vi "Configure controller.vi"(2 "Ti (s)":sgl=0.1, 3 "Kp":sgl=0.035, 4 "RPM":sgl(knob) min=-1000 max=1000 scale=-1000.0..1000.0, 5 "Set RPM only (else full config.)":bool) -> (0 "error out":errorcluster)   [LabVIEW 2015]
uses:
  Arduino_common/Arduino_comms_Global.vi
panel:
  in  "Device index":i32=1
  in  "Reset":bool
  in  "Control system configuration":enum32{"Encoder", "Motor", "RPM", "PID"}(tab)=enum."PID"
  in  "Encoder PPR":u16=256
  in  "Encoder x1/x2/x4":u8(ring)=1 items=["1"=1, "2"=2, "4"=4]
  in  "Vmotor_max":sgl=6.0
  in  "Vmotor_min":sgl=-6.0
  in  "Gearbox ratio (shaft : motor)":sgl=0.24561404
  in  "RPM_max":sgl=1000.0
  in  "RPM_min":sgl=-1000.0
  in  "RPM_tol":sgl
  in  "Td (s)":sgl
  out "Bytes sent":u32
  out "Write buffer":string
  # "Paul Nathan, 03/08/2013"
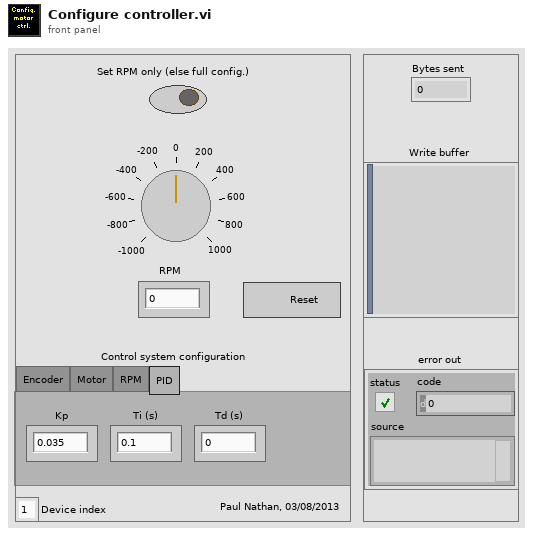
[diagram p1: front panel]
types:
  T1 = typedef "Arduino Config & resource typedef.ctl" = cluster{"VISA resource name":refnum<visa-resource-name>, "baud rate (bps)":u32, "timeout (ms)":u32, "data bits":u16, "parity":enum16{"None", "Odd", "Even", "Mark", "Space"}, "stop bits (10: 1 bit)":u16, "flow control":u16, "termination char (hex)":u8, "Enable Termination Char":bool, "byte count":u32, "Resource locked?":bool}
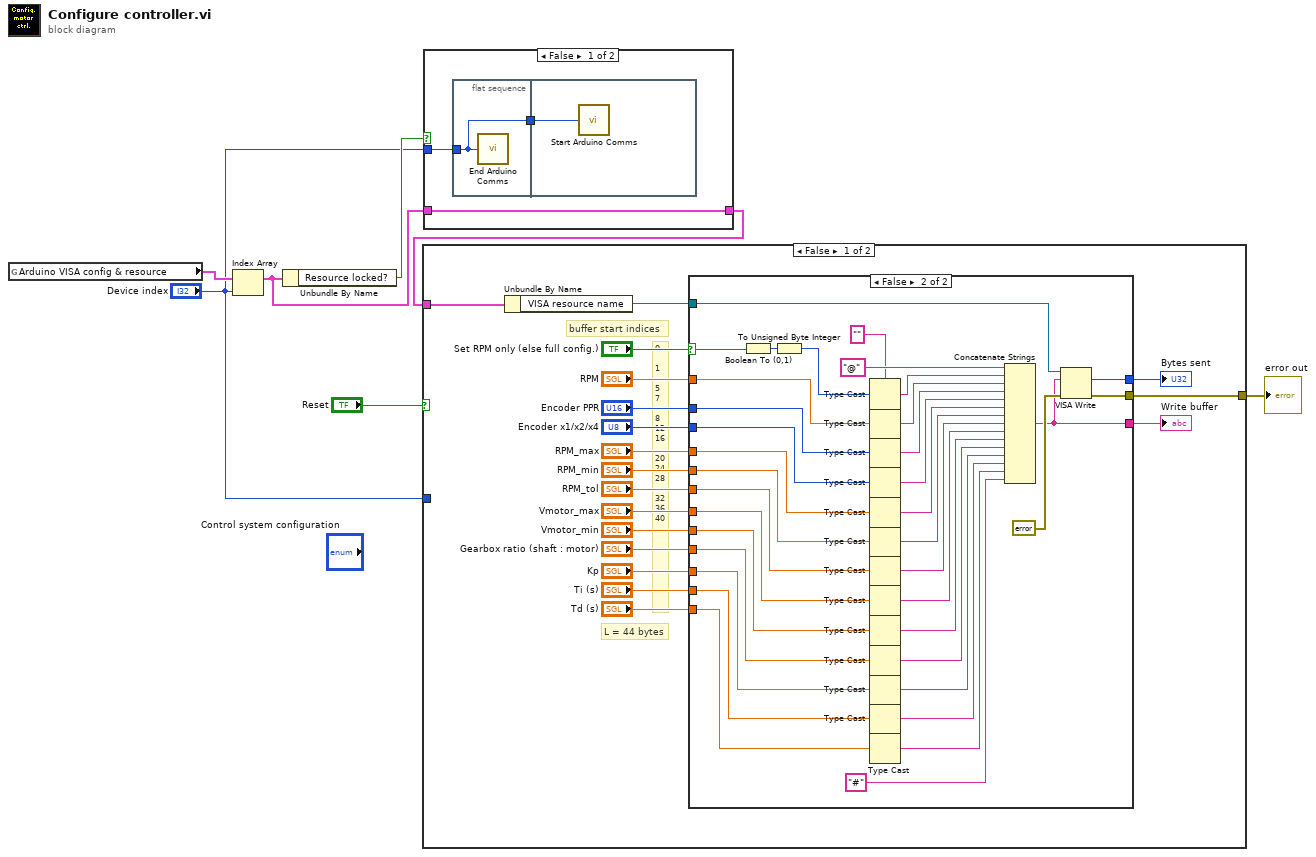
[diagram p0: block diagram]
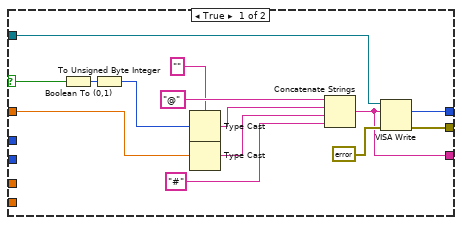
[diagram p3: hidden frame]
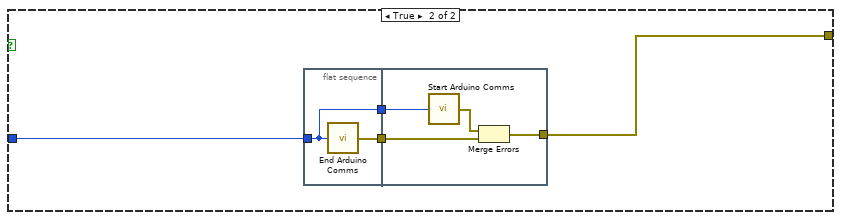
[diagram p4: hidden frame]
diagram:
  n1 = global read "Arduino_comms_Global.vi" "Arduino VISA config & resource"() -> (w5:T1[])
  n2 = Index Array(array=w5, index="Device index") -> (element=w3:T1)
  n3 = Unbundle By Name(w3) -> ("Resource locked?"=w6:bool)
  n4 = case shown="False" w6 {
    tunnel: w3 -> [w10 w13]
    tunnel: [w10 w13] -> w4
    tunnel: "Device index" -> [w9 _]
    frame False {
      n5 = flat-sequence {
        tunnel: w9 -> [w11]
        tunnel: [w11] -> w8
        tunnel: w8 -> [w12]
        frame #0 {
          n6 = call "End Arduino Comms.vi"("Resource index"=w11) -> ()  [unwired: 1 out]
        }
        frame #1 {
          n7 = call "Start Arduino Comms.vi"("Resource index"=w12) -> ()  [unwired: 1 out]
        }
      }
    }
    frame True {
    }
  }
  n8 = case shown="False" "Reset" {
    tunnel: [w30 w84] -> w1
    tunnel: w4 -> [w14 _]
    tunnel: "Device index" -> [_ w83]
    frame False {
      # "L = 44 bytes"
      # "buffer start indices"
      # "0\n\n1\n\n5\n7\n\n8\n12\n16\n\n20\n24\n28\n\n32\n36\n40"
      n9 = Unbundle By Name(w14) -> ("VISA resource name"=w31:refnum<visa-resource-name>)
      n10 = case shown="False" "Set RPM only (else full config.)" {
        selector: "Set RPM only (else full config.)" -> [w39 w75]
        tunnel: w31 -> [w45 w81]
        tunnel: [w44 w80] -> w30
        tunnel: "RPM" -> [w36 w72]
        tunnel: [w35 w70] -> w27
        tunnel: [w34 w71] -> w26
        tunnel: "Encoder PPR" -> [_ w58]
        tunnel: "Encoder x1/x2/x4" -> [_ w57]
        tunnel: "RPM_max" -> [_ w56]
        tunnel: "RPM_min" -> [_ w55]
        tunnel: "RPM_tol" -> [_ w54]
        tunnel: "Vmotor_max" -> [_ w53]
        tunnel: "Vmotor_min" -> [_ w52]
        tunnel: "Gearbox ratio (shaft : motor)" -> [_ w51]
        tunnel: "Kp" -> [_ w50]
        tunnel: "Ti (s)" -> [_ w49]
        tunnel: "Td (s)" -> [_ w48]
        frame True {
          w32 = ""
          n11 = Boolean To (0,1)(Boolean=w39) -> (0, 1=w38:i16)
          n12 = To Unsigned Byte Integer(number=w38) -> (unsigned 8bit integer=w37:u8)
          n13 = Type Cast(type=w32, x=w37) -> (*(type *) &x=w42:string)
          n14 = Type Cast(type=w32, x=w36) -> (*(type *) &x=w41:string)
          n15 = Concatenate Strings("@", w42, w41, "#") -> (w34:string)
          n16 = VISA Write(VISA resource name=w45, write buffer=w34, error in (no error)=errorcluster {"status"=FALSE, "code"=0, "source"=""}) -> (return count=w35:u32, error out=w44:errorcluster)  [unwired: 1 out]
        }
        frame False {
          w46 = ""
          n17 = Boolean To (0,1)(Boolean=w75) -> (0, 1=w74:i16)
          n18 = To Unsigned Byte Integer(number=w74) -> (unsigned 8bit integer=w73:u8)
          n19 = Type Cast(type=w46, x=w73) -> (*(type *) &x=w78:string)
          n20 = Type Cast(type=w46, x=w72) -> (*(type *) &x=w77:string)
          n21 = Type Cast(type=w46, x=w58) -> (*(type *) &x=w69:string)
          n22 = Type Cast(type=w46, x=w57) -> (*(type *) &x=w68:string)
          n23 = Type Cast(type=w46, x=w56) -> (*(type *) &x=w67:string)
          n24 = Type Cast(type=w46, x=w55) -> (*(type *) &x=w66:string)
          n25 = Type Cast(type=w46, x=w54) -> (*(type *) &x=w65:string)
          n26 = Type Cast(type=w46, x=w53) -> (*(type *) &x=w64:string)
          n27 = Type Cast(type=w46, x=w52) -> (*(type *) &x=w63:string)
          n28 = Type Cast(type=w46, x=w51) -> (*(type *) &x=w62:string)
          n29 = Type Cast(type=w46, x=w50) -> (*(type *) &x=w61:string)
          n30 = Type Cast(type=w46, x=w49) -> (*(type *) &x=w60:string)
          n31 = Type Cast(type=w46, x=w48) -> (*(type *) &x=w59:string)
          n32 = Concatenate Strings("@", w78, w77, w69, w68, w67, w66, w65, w64, w63, w62, w61, w60, w59, "#") -> (w71:string)
          n33 = VISA Write(VISA resource name=w81, write buffer=w71, error in (no error)=errorcluster {"status"=FALSE, "code"=0, "source"=""}) -> (return count=w70:u32, error out=w80:errorcluster)  [unwired: 1 out]
        }
      }
      "Write buffer" <- w26
      "Bytes sent" <- w27
    }
    frame True {
      n34 = flat-sequence {
        tunnel: [w87] -> w85
        tunnel: w83 -> [w86]
        tunnel: [w86] -> w82
        tunnel: [w88] -> w84
        tunnel: w85 -> [w89]
        tunnel: w82 -> [w91]
        frame #0 {
          n35 = call "End Arduino Comms.vi"("Resource index"=w86) -> ("Error"=w87:errorcluster)
        }
        frame #1 {
          n36 = call "Start Arduino Comms.vi"("Resource index"=w91) -> ("Error"=w90:errorcluster)
          n37 = Merge Errors(w90, w89) -> (w88:errorcluster)
        }
      }
    }
  }
  "error out" <- w1
